vi "ResistanceStatus.vi"(0 "TestIndex":i32, 1 "延时":u32=1000, 2 "索引 (列)":i32=4, 3 "error in (no error)":errorcluster caption="错误输入（无错误）", 4 "阀值":i32=1000) -> (5 "常灭":i32=8, 6 "结果":bool=TRUE, 7 "常亮":i32, 8 "灯数值数组":i32[][](array[numeric]), 9 "闪":i32, 10 "error out":errorcluster={"status"=FALSE, "code"=1073676294, "source"="ColorSensor.vi->ResistanceStatus.vi中的VISA读取"} caption="错误输出")   [LabVIEW 2015]
panel:
  out "大小":i32[](array[numeric])=[8, 8]
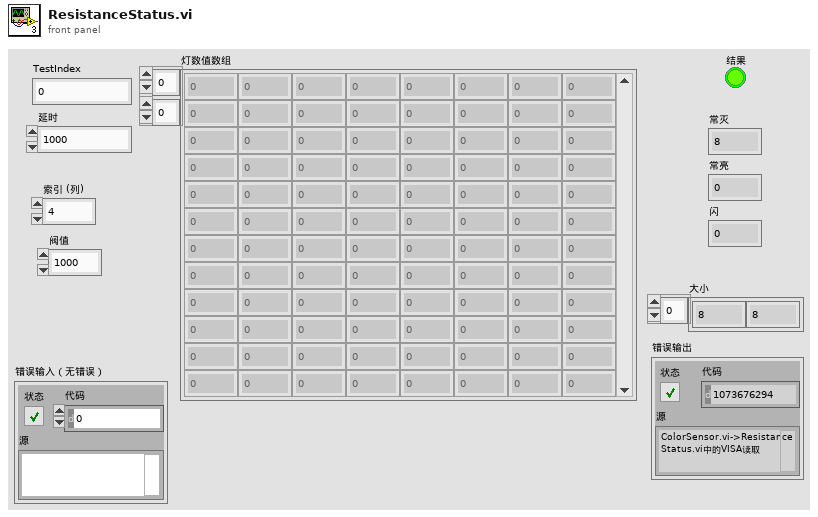
[diagram p1: front panel]
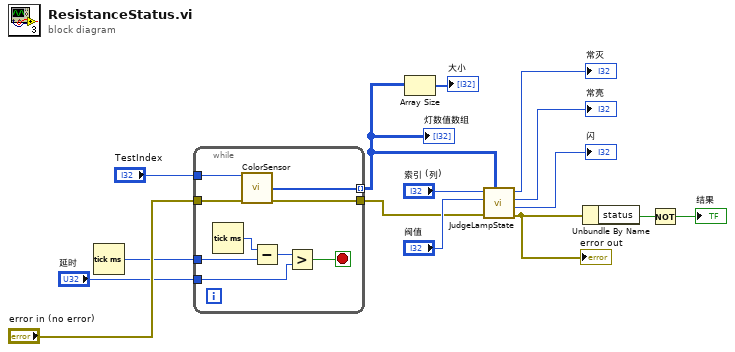
[diagram p0: block diagram]
diagram:
  n1 = Tick Count (ms)() -> (millisecond timer value=w13:u32)
  n2 = while {
    tunnel: "TestIndex" -> [w24]
    tunnel: "error in (no error)" -> [w23]
    tunnel: w13 -> [w21]
    tunnel: "延时" -> [w19]
    tunnel: [w17] -> w8 mode=indexing
    tunnel: [w16] -> w5
    stop <- w18 stop-if-true
    n3 = Tick Count (ms)() -> (millisecond timer value=w22:u32)
    n4 = call "ColorSensor.vi"("TestIndex"=w24, "error in (no error)"=w23) -> ("数值数组"=w17:i32[], "error out"=w16:errorcluster)  [unwired: 10 in, 2 out]
    n5 = Subtract(x=w22, y=w21) -> (x-y=w20:u32)
    n6 = Greater?(x=w20, y=w19) -> (0:w18:bool)
  }
  "灯数值数组" <- w8
  n7 = Array Size(array=w8) -> (size(s)=→"大小":i32[])
  n8 = call "JudgeLampState.vi"("数值数组"=w8, "error in (no error)"=w5, "阀值"="阀值", "灯索引 (列)"="索引 (列)") -> ("error out"=w4:errorcluster, "闪"=→"闪":i32, "常亮"=→"常亮":i32, "常灭"=→"常灭":i32)  [unwired: 4 in]
  "error out" <- w4
  n9 = Unbundle By Name(w4) -> ("status"=w11:bool)
  n10 = Not(x=w11) -> (.not. x?=→"结果":bool)
